vi "主程序.vi"() -> ()   [LabVIEW 2021]
uses:
  <vilib>/Utility/miscctls.llb/LVRowAndColumnTypeDef.ctl
  <vilib>/Utility/file.llb/Write Delimited Spreadsheet (string).vi
  <vilib>/Utility/file.llb/Read Delimited Spreadsheet (DBL).vi
  <instrlib>/Keithley DMM6500 DAQ6500 Series/Public/Data/Read (Single Point).vi
  <instrlib>/Keithley 27XX/Public/Data/Read Single Point.vi
  <vilib>/Utility/file.llb/Read Delimited Spreadsheet (string).vi
  <instrlib>/Keithley DMM6500 DAQ6500 Series/Keithley DMM6500 DAQ6500 Series.lvlib
  <instrlib>/Keithley 27XX/Keithley 27XX.lvlib
  <instrlib>/Keithley DMM7510/Keithley DMM7510.lvlib
panel:
  out "x*y":dbl
  in  "电压输出传感器精度":dbl(ring) items=["3‰"=0.003, "5‰"=0.005, "8‰"=0.008, "1％"=0.01, "5％"=0.05, "10％"=0.1]
  in  "量程2灵敏度":dbl(ring) items=["S12"=1.67, "S08"=2.5]
  in  "精度":dbl(ring) items=["3‰"=0.003, "5‰"=0.005, "8‰"=0.008, "1％"=0.01, "5％"=0.05, "10％"=0.1]
  out "?":bool
  in  "?":bool
  out "x != y?":bool
  in  "?":bool
  in  "SN":string
  in  "?":enum16{"CAB500", "CAB1500"}(ring)
  in  "电压读取":refnum<visa-resource-name>
  in  "仪器实例 out 4":T1
  in  "传感器缩放系数":dbl(ring) items=["2000"=2000.0, "5000"=5000.0]
  in  "量程1灵敏度":dbl(ring) items=["S12"=1.67, "S08"=2.5]
  out "?":bool
  in  "电流选择":u16(ring) items=["请选择", "5", "±100", "±200", "±300", "±50", "±500"]
  in  "?":bool
  in  "?":bool
  in  "电压输出电流传感器测试":i32(listbox)
  in  "电流传感器测试":i32(listbox)
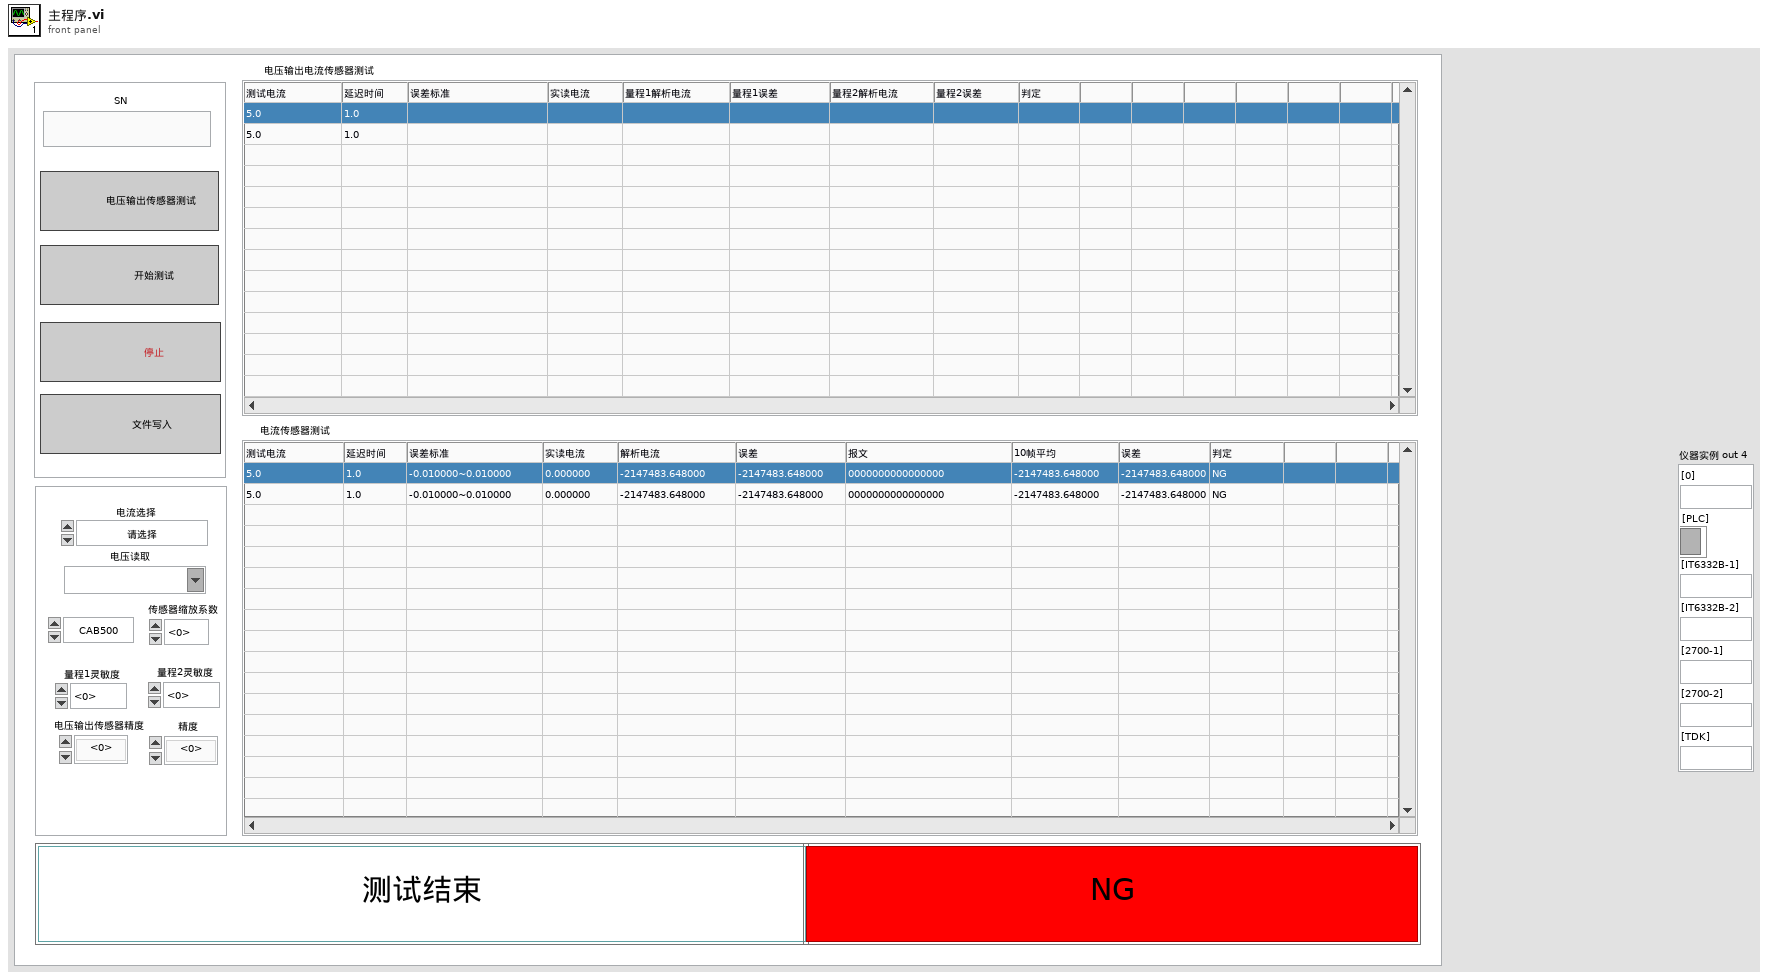
[diagram p1: front panel]
types:
  T1 = typedef "仪器实例.ctl" = cluster{"[0]":string, "[PLC]":refnum<k24>, "[IT6332B-1]":string, "[IT6332B-2]":string, "[2700-1]":string, "[2700-2]":string, "[TDK]":string}
  T2 = typedef "仪器地址输入.ctl" = cluster{"[PLC]":string, "[IT6332B-1]":string, "[IT6332B-2]":string, "[2700-1]":string, "[2700-2]":string, "[TDK]":string}
  T3 = enum16{"open", "replace", "create", "open or create", "replace or create", "replace or create with confirmation"}
  T4 = typedef "LVRowAndColumnTypeDef.ctl" = cluster{"Row":i32, "Column":i32}
  T5 = enum32{"Invalid", "Standard", "Closed", "Hidden", "Minimized", "Maximized"}
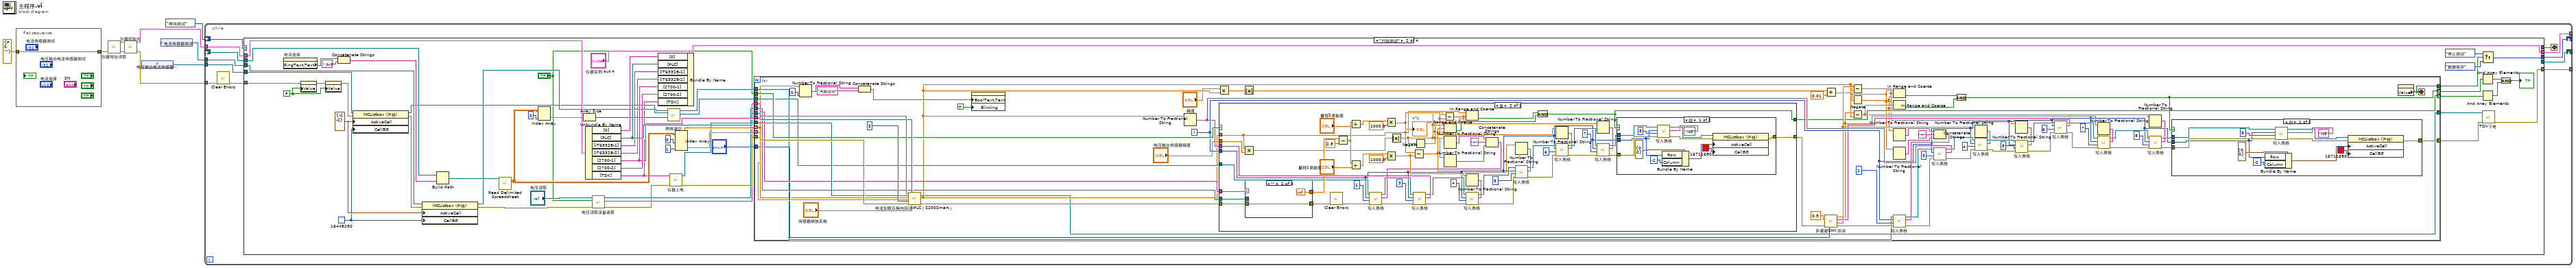
[diagram p0: block diagram]
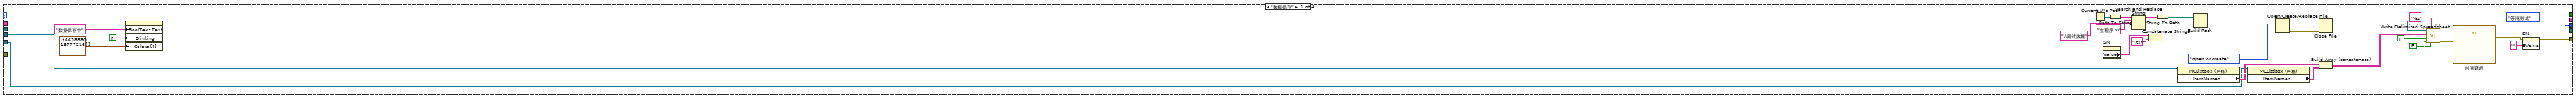
[diagram p2: hidden frame]
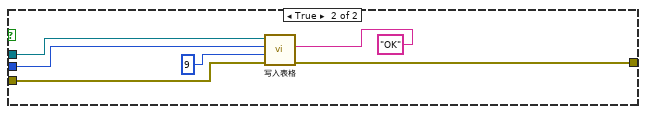
[diagram p3: hidden frame]
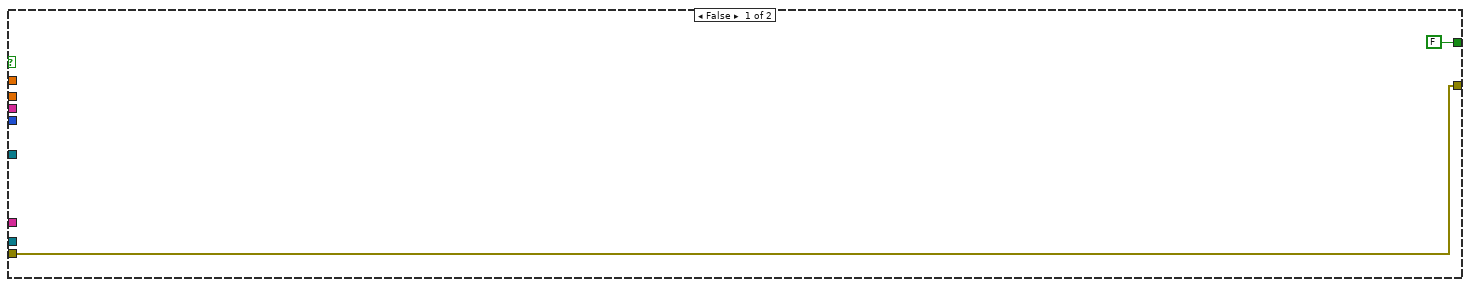
[diagram p4: hidden frame]
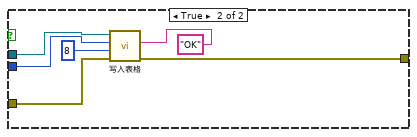
[diagram p5: hidden frame]
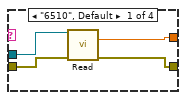
[diagram p6: hidden frame]
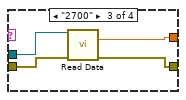
[diagram p7: hidden frame]
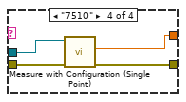
[diagram p8: hidden frame]
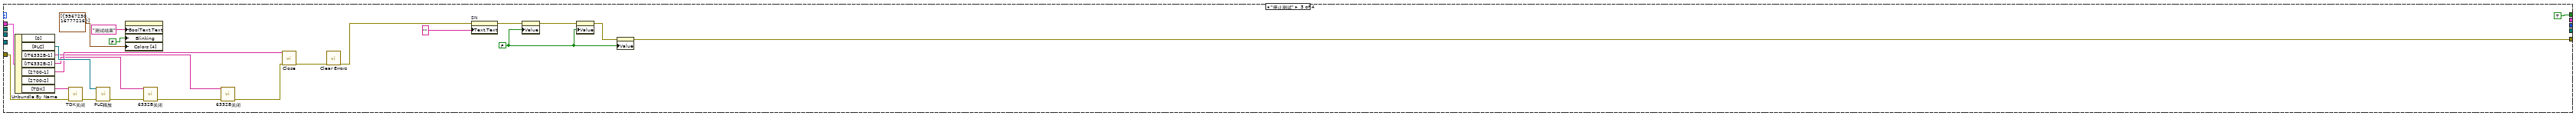
[diagram p9: hidden frame]
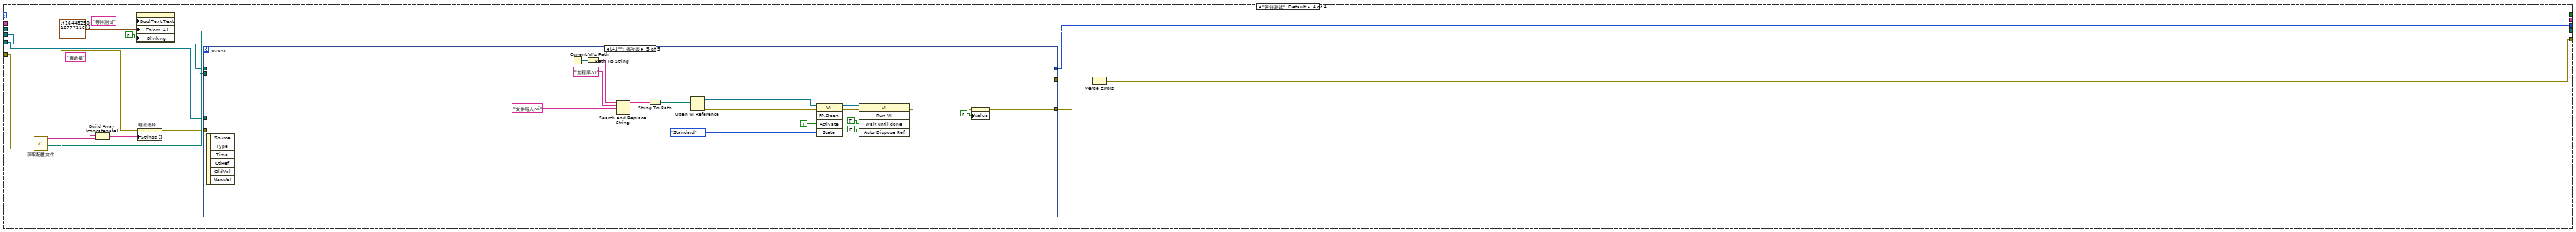
[diagram p10: hidden frame]
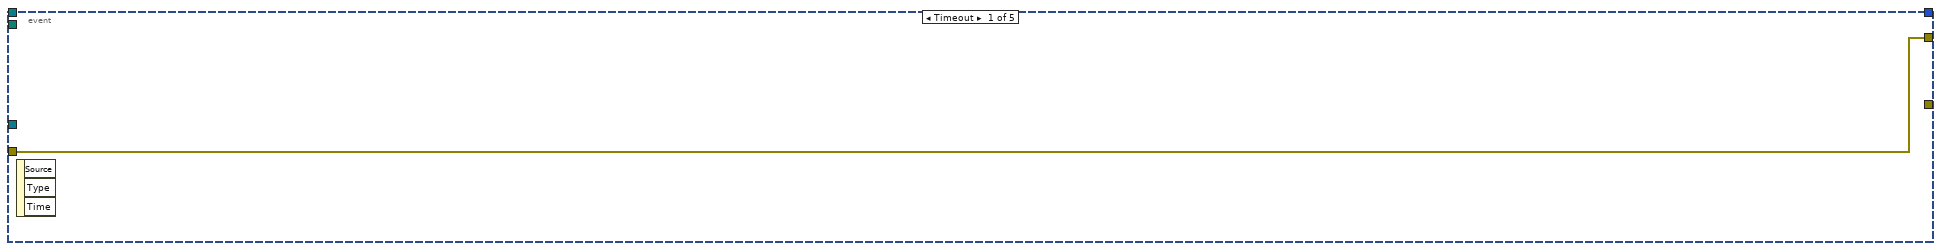
[diagram p11: hidden frame]
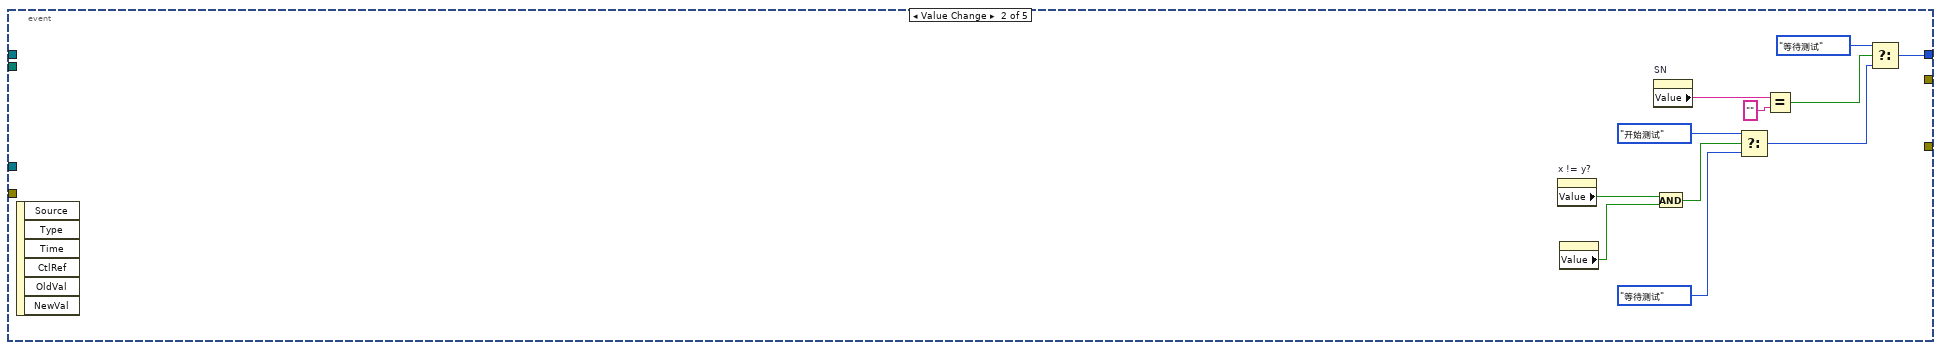
[diagram p12: hidden frame]
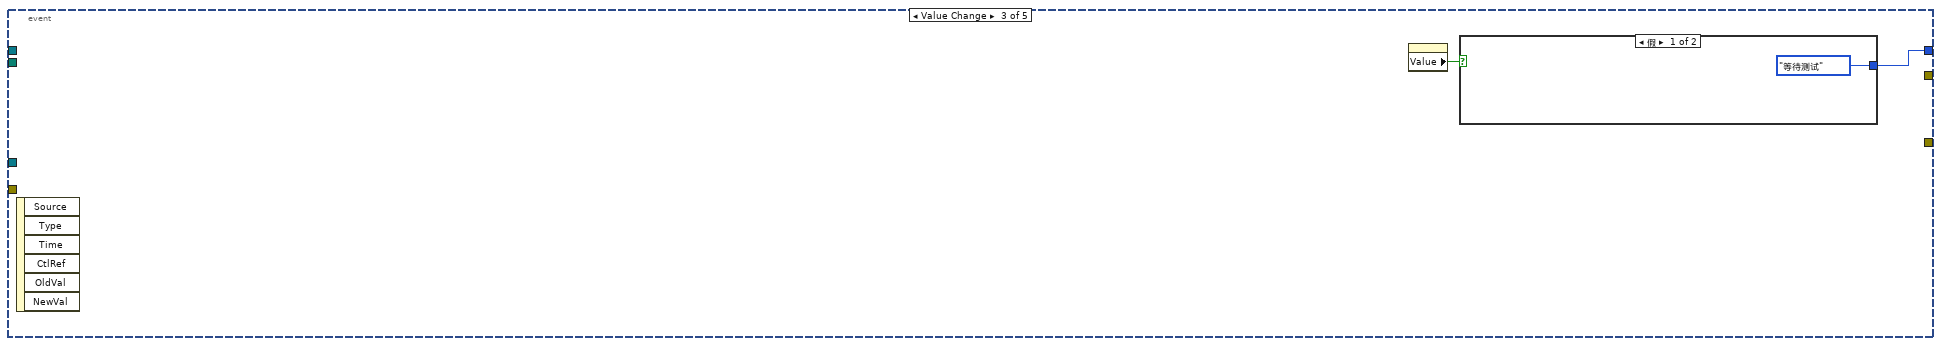
[diagram p13: hidden frame]
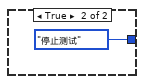
[diagram p14: hidden frame]
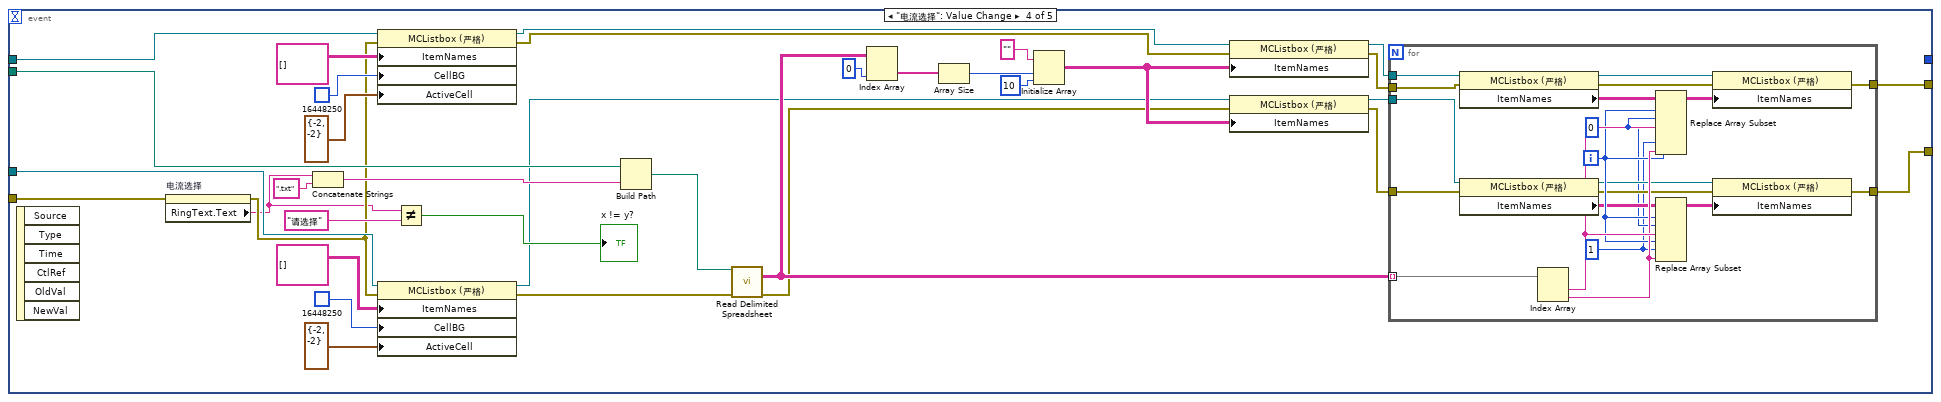
[diagram p15: hidden frame]
diagram:
  n1 = flat-sequence {
    tunnel: errorcluster {"status"=FALSE, "code"=0, "source"=""} ("error in (no error)") -> [w10]
    tunnel: [w10] -> w1
    frame #0 {
    }
  }
  n2 = call "仪器地址读取.vi"("error in (no error)"=w1) -> ("error out"=w9:errorcluster, "仪器地址"=w8:T2)  [unwired: 7 in]
  n3 = call "仪器初始化.vi"("错误输入（无错误）"=w9, "仪器地址"=w8) -> ("error out"=w6:errorcluster, "仪器实例 out"=w5:T1)  [unwired: 8 in]
  n4 = control-ref of="电压输出电流传感器测试"() -> (w3:refnum<vi>)
  n5 = control-ref of="电流传感器测试"() -> (w4:refnum<vi>)
  n6 = while {
    shift-right: [w21] -> _
    shift-left: enum16{"等待测试", "开始测试", "停止测试", "数据保存"}."等待测试" -> [w22]
    shift-right: [w17] -> _
    shift-left: _ -> [w16]
    tunnel: w3 -> [w12]
    tunnel: w4 -> [w11]
    tunnel: w5 -> [w19]
    tunnel: [w20] -> _
    tunnel: w6 -> [w14]
    tunnel: [w18] -> _
    stop <- w15 stop-if-true
    n7 = call <vilib>:"Clear Errors.vi"("error in (no error)"=w14) -> ("error out"=w13:errorcluster)  [unwired: 5 in, 1 out]
    n8 = case shown="\"开始测试\"" w22 {
      tunnel: [enum16{"等待测试", "开始测试", "停止测试", "数据保存"}."等待测试" w74 _ w319] -> w21
      tunnel: w19 -> [_ w102 w316 _]
      tunnel: w13 -> [_ w79 w312 w324]
      tunnel: [_ w101 _ _] -> w20
      tunnel: [w32 w63 w296 w325] -> w18
      tunnel: [_ _ _ w322] -> w17
      tunnel: w16 -> [_ w97 _ _]
      tunnel: [_ _ TRUE _] -> w15
      tunnel: w11 -> [w36 w89 _ w320]
      tunnel: w12 -> [w35 w90 _ w321]
      frame "数据保存" {
        n9 = property class="Bool (严格)"("BoolText.Text"="数据保存中" ("布尔文本.文本"), "Blinking"=FALSE ("闪烁"), "Colors [4]"=cluster{u32, u32}[] [{6618880, 16777216}] ("颜色[4]")) -> ()  [unwired: 2 in, 2 out]
        n10 = Current VI's Path() -> (path=w27:path)
        n11 = property on="SN" class="Str"() -> ("Value"=w34:string)  [unwired: 2 in, 2 out]
        n12 = Path To String(path=w27) -> (string=w25:string)
        n13 = Search and Replace String(input string=w25, search string="主程序.vi" ("搜索字符串"), replace string="\\测试数据" ("字符串")) -> (result string=w23:string)  [unwired: 5 in, 3 out]
        n14 = Concatenate Strings(w34, ".txt" ("字符串")) -> (w43:string)
        n15 = String To Path(string=w23) -> (path=w28:path)
        n16 = property class="MCListbox (严格)"(reference=w36) -> (error out=w54:errorcluster, "ItemNames"=w53:string[][])  [unwired: 1 in, 1 out]
        n17 = Build Path(base path=w28, name or relative path=w43) -> (appended path=w40:path)
        n18 = property class="MCListbox (严格)"(reference=w35, error in=w54) -> (error out=w48:errorcluster, "ItemNames"=w52:string[][])  [unwired: 1 out]
        n19 = Open/Create/Replace File(file path (use dialog)=w40, operation (0:open)=T3."open or create" ("操作(0:open)")) -> (refnum out=w42:refnum<file>, error out=w45:errorcluster)  [unwired: 4 in, 1 out]
        n20 = Close File(refnum=w42, error in=w45) -> (path=w39:path)  [unwired: 1 out]
        n21 = Build Array (concatenate)(w53, w52) -> (w51:string[][])
        n22 = call-poly <vilib>:"Write Delimited Spreadsheet.vi"("file path (dialog if empty)"=w39, "format (%s)"="%s", "2D data"=w51, "append to file? (new file:F)"=TRUE, "error in (no error)"=w48, "transpose? (no:F)"=FALSE) -> ("error out"=w30:errorcluster)  [unwired: 8 in, 1 out]
        n23 = call "时间延迟"("error in (no error)"=w30) -> ("error out"=w29:errorcluster)  [unwired: 10 in]
        n24 = property on="SN" class="Str"(error in=w29, "Value"="" ("SN")) -> (error out=w32:errorcluster)  [unwired: 1 in, 1 out]
      }
      frame "开始测试" {
        w81 = FALSE
        w92 = T4 {"Row"=-2, "Column"=-2} ("活动单元格:活动单元格")
        w91 = u32 16448250
        n25 = property on="电流选择" class="Ring (严格)"() -> ("RingText.Text"=w100:string)  [unwired: 2 in, 2 out]
        n26 = property class="Bool (严格)"(error in=w79, "Value"=w81) -> (error out=w82:errorcluster)  [unwired: 1 in, 1 out]
        n27 = property class="Bool (严格)"(error in=w82, "Value"=w81) -> (error out=w80:errorcluster)  [unwired: 1 in, 1 out]
        n28 = Concatenate Strings(w100, ".txt" ("字符串")) -> (w98:string)
        n29 = property class="MCListbox (严格)"(reference=w90, error in=w80, "ActiveCell"=w92, "CellBG"=w91) -> (reference out=w69:refnum<vi>, error out=w93:errorcluster)
        n30 = property class="MCListbox (严格)"(reference=w89, error in=w93, "ActiveCell"=w92, "CellBG"=w91) -> (reference out=w70:refnum<vi>, error out=w59:errorcluster)
        n31 = Build Path(base path=w97, name or relative path=w98) -> (appended path=w96:path)
        n32 = call-poly <vilib>:"Read Delimited Spreadsheet.vi"("file path (dialog if empty)"=w96) -> ("all rows"=w85:dbl[][])  [unwired: 9 in, 5 out]
        n33 = Index Array(array=w85, index (col)=0 ("禁用的索引 (列)")) -> (element=w83:dbl[])  [unwired: 1 in]
        n34 = Array Size(array=w83) -> (size(s)=w71:i32)
        n35 = Unbundle By Name(w102) -> ("[0]"=w105:string, "[PLC]"=w75:refnum<k24>, "[IT6332B-1]"=w55:string, "[IT6332B-2]"=w66:string, "[2700-1]"=w106:string, "[2700-2]"=w107:string, "[TDK]"=w67:string)
        n36 = call "电压读取设备选取.vi"("error out"=w59, "布尔"="?", "电压读取"="电压读取") -> ("error out 2"=w56:errorcluster, "所有匹配"=w57:string, "VISA resource name out"=w58:refnum<visa-resource-name>)  [unwired: 6 in]
        n37 = Bundle By Name(cluster="仪器实例 out 4", "[0]"=w105, "[PLC]"=w75, "[IT6332B-1]"=w55, "[IT6332B-2]"=w66, "[2700-1]"=w106, "[2700-2]"=w107, "[TDK]"=w67) -> (w101:T1)
        n38 = call "表格清空.vi"("数值"=w71, "电压输出电流传感器测试"=w69, "电流传感器测试"=w70) -> ("电压输出电流传感器测试 2"=w72:refnum<vi>, "电流传感器测试 2"=w73:refnum<vi>)  [unwired: 7 in]
        n39 = call "仪器上电.vi"("错误输入"=w56, "VISA resource name"=w67) -> ("error out"=w65:errorcluster, "VISA resource name out"=w68:refnum<visa-resource-name>)  [unwired: 8 in]
        n40 = Index Array(array=w85, index (col) #1=0 ("禁用的索引 (列)"), index (col) #2=1 ("索引 (列)")) -> (element #1=w110:dbl[], element #2=w109:dbl[])  [unwired: 2 in]
        n41 = for {
          tunnel: w68 -> [w181]
          tunnel: w65 -> [w185]
          tunnel: [w152] -> w64
          tunnel: w110 -> [w128] mode=indexing
          tunnel: w109 -> [w183] mode=indexing
          tunnel: w106 -> [w182]
          tunnel: w75 -> [w179]
          tunnel: w57 -> [w178]
          tunnel: w58 -> [w177]
          tunnel: "?" -> [w175]
          tunnel: "?" -> [w141]
          tunnel: w73 -> [w137]
          tunnel: w72 -> [w151]
          tunnel: [w130] -> w78 mode=indexing
          tunnel: [w129] -> w88 mode=indexing
          tunnel: [w123] -> w76
          tunnel: [w121] -> w62
          i -> [w145]
          stop <- w123 stop-if-true
          n42 = Number To Fractional String(number=w128, precision (6)=i16 0 ("精度(6)")) -> (F-format string=w132:string)  [unwired: 2 in]
          n43 = Concatenate Strings(w132, "A测试中" ("字符串")) -> (w135:string)
          n44 = call "电流加载及换向回读-PLC（S200Smart）.vi"("6510 in"=w182, "TDK in"=w181, "输入电流"=w128, "Delay Time (s)"=w183, "电源台数"=u8 3, "error in"=w185, "引用输出"=w179, "y"="传感器缩放系数") -> ("TDK out"=w121:refnum<visa-resource-name>, "实际电流"=w127:dbl, "error out"=w176:errorcluster)  [unwired: 8 in, 1 out]
          n45 = property class="Bool (严格)"("BoolText.Text"=w135, "Blinking"=TRUE ("闪烁")) -> ()  [unwired: 2 in, 2 out]
          n46 = Number To Fractional String(number=w127) -> (F-format string=w153:string)  [unwired: 3 in]
          n47 = Multiply(x="精度", y=w127) -> (x*y=w112:dbl)
          n48 = case shown="真" w175 {
            tunnel: w178 -> [_ w261]
            tunnel: w177 -> [_ w260]
            tunnel: w176 -> [w205 w259]
            tunnel: [w205 w224] -> w143
            tunnel: w153 -> [_ w253]
            tunnel: w145 -> [_ w225]
            tunnel: w127 -> [_ w220]
            tunnel: w151 -> [_ w232]
            tunnel: [FALSE w215] -> w129
            tunnel: "电压输出传感器精度" -> [_ w213]
            frame False {
            }
            frame True {
              n49 = Multiply(x=w220, y=w213) -> (x*y=w208:dbl)
              n50 = case shown="\"\"" w261 {
                tunnel: w260 -> [w283 _ w289 w290]
                tunnel: w259 -> [w281 w285 w287 w293]
                tunnel: [w280 w285 w286 w292] -> w241
                tunnel: [w282 inf w288 w291] -> w258
                frame "6510", Default {
                  n51 = call-poly <instrlib>:"Read.vi"("VISA resource name"=w283, "error in (no error)"=w281) -> ("Measurement"=w282:dbl, "error out"=w280:errorcluster)  [unwired: 11 in, 1 out]
                }
                frame "" {
                }
                frame "2700" {
                  n52 = call-poly <instrlib>:"Read Data.vi"("VISA resource name"=w289, "error in (no error)"=w287) -> ("Measurement Data"=w288:dbl, "error out"=w286:errorcluster)  [unwired: 11 in, 1 out]
                }
                frame "7510" {
                  n53 = call <instrlib>:"Measure with Configuration (Single Point).vi"("error in (no error)"=w293, "VISA resource name"=w290) -> ("error out"=w292:errorcluster, "Measurement"=w291:dbl)  [unwired: 6 in, 2 out]
                }
              }
              n54 = call <vilib>:"Clear Errors.vi"("error in (no error)"=w241) -> ("error out"=w235:errorcluster)  [unwired: 5 in, 1 out]
              n55 = Subtract(x=w258, y=2.5) -> (x-y=w222:dbl)
              n56 = Divide(x=w222, y="量程2灵敏度") -> (x/y=w219:dbl)
              n57 = Divide(x=w222, y="量程1灵敏度") -> (x/y=w255:dbl)
              n58 = Multiply(x=w219, y=1000.0) -> (x*y=w217:dbl)
              "x*y" <- w217
              n59 = Multiply(x=w255, y=1000.0) -> (x*y=w244:dbl)
              n60 = Absolute Value(x=w208) -> (abs(x)=w207:dbl)
              n61 = Subtract(x=w220, y=w244) -> (x-y=w209:dbl)
              n62 = Negate(x=w207) -> (-x=w206:dbl)
              n63 = Subtract(x=w220, y=w217) -> (x-y=w211:dbl)
              n64 = In Range and Coerce(upper limit=w207, x=w209, lower limit=w206) -> (In Range?=w212:bool)  [unwired: 1 out]
              n65 = Number To Fractional String(number=w206) -> (F-format string=w229:string)  [unwired: 3 in]
              n66 = Number To Fractional String(number=w207) -> (F-format string=w228:string)  [unwired: 3 in]
              n67 = In Range and Coerce(upper limit=w207, x=w211, lower limit=w206) -> (In Range?=w210:bool)  [unwired: 1 out]
              n68 = Number To Fractional String(number=w244) -> (F-format string=w249:string)  [unwired: 3 in]
              n69 = Concatenate Strings(w229, "~" ("字符串"), w228) -> (w227:string)
              n70 = call "写入表格.vi"("新元素/子数组"=w227, "错误输入（无错误）"=w235, "禁用的索引 (列)"=2, "索引 (行)"=w225, "引用"=w232) -> ("错误输出"=w234:errorcluster, "引用输出"=w231:refnum<vi>)  [unwired: 5 in]
              n71 = call "写入表格.vi"("新元素/子数组"=w253, "错误输入（无错误）"=w234, "禁用的索引 (列)"=3, "索引 (行)"=w225, "引用"=w231) -> ("错误输出"=w251:errorcluster, "引用输出"=w248:refnum<vi>)  [unwired: 5 in]
              n72 = call "写入表格.vi"("新元素/子数组"=w249, "错误输入（无错误）"=w251, "禁用的索引 (列)"=4, "索引 (行)"=w225, "引用"=w248) -> ("错误输出"=w250:errorcluster, "引用输出"=w247:refnum<vi>)  [unwired: 5 in]
              n73 = Number To Fractional String(number=w209) -> (F-format string=w243:string)  [unwired: 3 in]
              n74 = call "写入表格.vi"("新元素/子数组"=w243, "错误输入（无错误）"=w250, "禁用的索引 (列)"=5, "索引 (行)"=w225, "引用"=w247) -> ("错误输出"=w240:errorcluster, "引用输出"=w237:refnum<vi>)  [unwired: 5 in]
              n75 = And(x=w210, y=w212) -> (x .and. y?=w215:bool)
              n76 = Number To Fractional String(number=w217) -> (F-format string=w221:string)  [unwired: 3 in]
              n77 = call "写入表格.vi"("新元素/子数组"=w221, "错误输入（无错误）"=w240, "禁用的索引 (列)"=6, "索引 (行)"=w225, "引用"=w237) -> ("错误输出"=w239:errorcluster, "引用输出"=w236:refnum<vi>)  [unwired: 5 in]
              n78 = Number To Fractional String(number=w211) -> (F-format string=w216:string)  [unwired: 3 in]
              n79 = call "写入表格.vi"("新元素/子数组"=w216, "错误输入（无错误）"=w239, "禁用的索引 (列)"=7, "索引 (行)"=w225, "引用"=w236) -> ("错误输出"=w223:errorcluster, "引用输出"=w226:refnum<vi>)  [unwired: 5 in]
              n80 = case shown="假" w215 {
                tunnel: w223 -> [w272 w279]
                tunnel: [w267 w276] -> w224
                tunnel: w226 -> [w263 w275]
                tunnel: w225 -> [w262 w274]
                frame False {
                  n81 = call "写入表格.vi"("新元素/子数组"="NG", "错误输入（无错误）"=w272, "禁用的索引 (列)"=8, "索引 (行)"=w262, "引用"=w263) -> ("错误输出"=w268:errorcluster, "引用输出"=w271:refnum<vi>)  [unwired: 5 in]
                  n82 = Bundle By Name(cluster=T4 {"Row"=0, "Column"=0} ("活动单元格:活动单元格"), "Row"=w262, "Column"=-2) -> (w269:T4)
                  n83 = property class="MCListbox (严格)"(reference=w271, error in=w268, "ActiveCell"=w269, "CellBG"=u32 16711680) -> (error out=w267:errorcluster)  [unwired: 1 out]
                }
                frame True {
                  n84 = call "写入表格.vi"("新元素/子数组"="OK", "错误输入（无错误）"=w279, "禁用的索引 (列)"=8, "索引 (行)"=w274, "引用"=w275) -> ("错误输出"=w276:errorcluster)  [unwired: 5 in, 1 out]
                }
              }
            }
          }
          n85 = Absolute Value(x=w112) -> (abs(x)=w113:dbl)
          n86 = call "多通道CAN 回读.vi"("传感器选择"=w141, "错误输入（无错误）"=w143, "Delay Time (s)"=0.5) -> ("错误输出"=w138:errorcluster, "解析电流"=w140:dbl, "报文数组"=w125:string, "十次平均"=w139:dbl)  [unwired: 5 in]
          n87 = Add(x=w113, y=0.01) -> (x+y=w116:dbl)
          n88 = Subtract(x=w140, y=w127) -> (x-y=w117:dbl)
          n89 = Negate(x=w116) -> (-x=w115:dbl)
          n90 = Subtract(x=w139, y=w127) -> (x-y=w119:dbl)
          n91 = In Range and Coerce(upper limit=w116, x=w117, lower limit=w115) -> (In Range?=w114:bool)  [unwired: 1 out]
          n92 = In Range and Coerce(upper limit=w116, x=w119, lower limit=w115) -> (In Range?=w118:bool)  [unwired: 1 out]
          n93 = Number To Fractional String(number=w115) -> (F-format string=w147:string)  [unwired: 3 in]
          n94 = Number To Fractional String(number=w116) -> (F-format string=w149:string)  [unwired: 3 in]
          n95 = Concatenate Strings(w147, "~" ("字符串"), w149) -> (w146:string)
          n96 = call "写入表格.vi"("新元素/子数组"=w146, "错误输入（无错误）"=w138, "禁用的索引 (列)"=2, "索引 (行)"=w145, "引用"=w137) -> ("错误输出"=w150:errorcluster, "引用输出"=w136:refnum<vi>)  [unwired: 5 in]
          n97 = call "写入表格.vi"("新元素/子数组"=w153, "错误输入（无错误）"=w150, "禁用的索引 (列)"=3, "索引 (行)"=w145, "引用"=w136) -> ("错误输出"=w167:errorcluster, "引用输出"=w174:refnum<vi>)  [unwired: 5 in]
          n98 = And(x=w114, y=w118) -> (x .and. y?=w130:bool)
          n99 = Number To Fractional String(number=w140) -> (F-format string=w168:string)  [unwired: 3 in]
          n100 = call "写入表格.vi"("新元素/子数组"=w168, "错误输入（无错误）"=w167, "禁用的索引 (列)"=4, "索引 (行)"=w145, "引用"=w174) -> ("错误输出"=w166:errorcluster, "引用输出"=w173:refnum<vi>)  [unwired: 5 in]
          n101 = Number To Fractional String(number=w117) -> (F-format string=w160:string)  [unwired: 3 in]
          n102 = call "写入表格.vi"("新元素/子数组"=w160, "错误输入（无错误）"=w166, "禁用的索引 (列)"=5, "索引 (行)"=w145, "引用"=w173) -> ("错误输出"=w165:errorcluster, "引用输出"=w172:refnum<vi>)  [unwired: 5 in]
          n103 = call "写入表格.vi"("新元素/子数组"=w125, "错误输入（无错误）"=w165, "禁用的索引 (列)"=6, "索引 (行)"=w145, "引用"=w172) -> ("错误输出"=w164:errorcluster, "引用输出"=w163:refnum<vi>)  [unwired: 5 in]
          n104 = Number To Fractional String(number=w139) -> (F-format string=w162:string)  [unwired: 3 in]
          n105 = call "写入表格.vi"("新元素/子数组"=w162, "错误输入（无错误）"=w164, "禁用的索引 (列)"=7, "索引 (行)"=w145, "引用"=w163) -> ("错误输出"=w159:errorcluster, "引用输出"=w156:refnum<vi>)  [unwired: 5 in]
          n106 = Number To Fractional String(number=w119) -> (F-format string=w157:string)  [unwired: 3 in]
          n107 = call "写入表格.vi"("新元素/子数组"=w157, "错误输入（无错误）"=w159, "禁用的索引 (列)"=8, "索引 (行)"=w145, "引用"=w156) -> ("错误输出"=w155:errorcluster, "引用输出"=w154:refnum<vi>)  [unwired: 5 in]
          n108 = case shown="假" w130 {
            tunnel: w155 -> [w196 w203]
            tunnel: w154 -> [w195 w202]
            tunnel: w145 -> [w187 w200]
            tunnel: [w190 w198] -> w152
            frame False {
              n109 = Bundle By Name(cluster=T4 {"Row"=0, "Column"=0} ("活动单元格:活动单元格"), "Row"=w187, "Column"=-2) -> (w192:T4)
              n110 = call "写入表格.vi"("新元素/子数组"="NG", "错误输入（无错误）"=w196, "禁用的索引 (列)"=9, "索引 (行)"=w187, "引用"=w195) -> ("错误输出"=w191:errorcluster, "引用输出"=w194:refnum<vi>)  [unwired: 5 in]
              n111 = property class="MCListbox (严格)"(reference=w194, error in=w191, "ActiveCell"=w192, "CellBG"=u32 16711680) -> (error out=w190:errorcluster)  [unwired: 1 out]
            }
            frame True {
              n112 = call "写入表格.vi"("新元素/子数组"="OK", "错误输入（无错误）"=w203, "禁用的索引 (列)"=9, "索引 (行)"=w200, "引用"=w202) -> ("错误输出"=w198:errorcluster)  [unwired: 5 in, 1 out]
            }
          }
          n113 = property class="Bool (严格)"() -> ("Value"=w123:bool)  [unwired: 2 in, 2 out]
        }
        n114 = And Array Elements(Boolean array=w78) -> (logical AND=w87:bool)
        n115 = And Array Elements(Boolean array=w88) -> (logical AND=w86:bool)
        n116 = Select(t=enum16{"等待测试", "开始测试", "停止测试", "数据保存"}."停止测试", s=w76, f=enum16{"等待测试", "开始测试", "停止测试", "数据保存"}."数据保存") -> (s? t:f=w74:enum16{"等待测试", "开始测试", "停止测试", "数据保存"})
        n117 = call "TDK下电.vi"("error in (no error)"=w64, "VISA resource name"=w62) -> ("error out"=w63:errorcluster)  [unwired: 8 in, 1 out]
        n118 = And(x=w87, y=w86) -> (x .and. y?=→"?":bool)
      }
      frame "停止测试" {
        w300 = FALSE
        n119 = Unbundle By Name(w316) -> ("[PLC]"=w314:refnum<k24>, "[IT6332B-1]"=w306:string, "[IT6332B-2]"=w309:string, "[2700-1]"=w311:string, "[TDK]"=w315:string)  [unwired: 2 out]
        n120 = call "TDK关闭.vi"("error in (no error)"=w312, "VISA resource name"=w315) -> ("error out"=w313:errorcluster)  [unwired: 9 in]
        n121 = call "PLC释放.vi"("错误输入（无错误） 2"=w313, "引用"=w314) -> ("错误输入（无错误）"=w307:errorcluster)  [unwired: 9 in]
        n122 = property class="Bool (严格)"("BoolText.Text"="测试结束" ("布尔文本.文本"), "Blinking"=FALSE ("闪烁"), "Colors [4]"=cluster{u32, u32}[] [{9567230, 16777216}] ("颜色[4]")) -> ()  [unwired: 2 in, 2 out]
        n123 = call "6332B关闭.vi"("错误输入"=w307, "VISA资源名称"=w309) -> ("error out"=w308:errorcluster)  [unwired: 9 in]
        n124 = call "6332B关闭.vi"("错误输入"=w308, "VISA资源名称"=w306) -> ("error out"=w305:errorcluster)  [unwired: 9 in]
        n125 = call <instrlib>:"Close.vi"("VISA resource name"=w311, "error in (no error)"=w305) -> ("error out"=w295:errorcluster)  [unwired: 13 in]
        n126 = call <vilib>:"Clear Errors.vi"("error in (no error)"=w295) -> ("error out"=w294:errorcluster)  [unwired: 5 in, 1 out]
        n127 = property on="SN" class="Str"(error in=w294, "Text.Text"="" ("文本.文本")) -> (error out=w301:errorcluster)  [unwired: 1 in, 1 out]
        n128 = property class="Bool (严格)"(error in=w301, "Value"=w300) -> (error out=w303:errorcluster)  [unwired: 1 in, 1 out]
        n129 = property class="Bool (严格)"(error in=w303, "Value"=w300) -> (error out=w299:errorcluster)  [unwired: 1 in, 1 out]
        n130 = property class="Bool (严格)"(error in=w299, "Value"=w300) -> (error out=w296:errorcluster)  [unwired: 1 in, 1 out]
      }
      frame "等待测试", Default {
        n131 = call "获取配置文件.vi"("错误输入"=w324) -> ("错误输出"=w323:errorcluster, "路径输出"=w322:path, "数组"=w332:string[])  [unwired: 8 in]
        n132 = Build Array (concatenate)("请选择", w332) -> (w331:string[])
        n133 = property class="Bool (严格)"("BoolText.Text"="等待测试" ("布尔文本.文本"), "Colors [4]"=cluster{u32, u32}[] [{16448250, 16777216}] ("颜色[4]"), "Blinking"=FALSE ("闪烁")) -> ()  [unwired: 2 in, 2 out]
        n134 = property on="电流选择" class="Ring (严格)"(error in=w323, "Strings []"=w331) -> (error out=w317:errorcluster)  [unwired: 1 in, 1 out]
        n135 = event shown="[4] \"\": 值改变" {
          selector: _ -> [_ _ _ _ _]
          dyn-events: _ -> [_ _ _ _ _]
          timeout: _ -> [_ _ _ _ _]
          tunnel: [w333 _ _ w376 _] -> w327
          tunnel: [_ _ _ w375 w411] -> w326
          tunnel: w320 -> [_ _ _ w360 _]
          tunnel: w321 -> [_ _ _ w355 _]
          tunnel: w322 -> [_ _ _ w370 _]
          tunnel: [_ w337 w346 _ _] -> w319
          tunnel: w317 -> [w333 _ _ w351 _]
          event Timeout {
            n136 = event-data() -> ()  [unwired: 1 in, 3 out]
          }
          event Value Change {
            n137 = event-data() -> ()  [unwired: 1 in, 6 out]
            n138 = property on="x != y?" class="Bool (严格)"() -> ("Value"=w343:bool)  [unwired: 2 in, 2 out]
            n139 = property class="Bool (严格)"() -> ("Value"=w342:bool)  [unwired: 2 in, 2 out]
            n140 = property on="SN" class="Str"() -> ("Value"=w336:string)  [unwired: 2 in, 2 out]
            n141 = And(x=w343, y=w342) -> (x .and. y?=w344:bool)
            n142 = Select(t=enum16{"等待测试", "开始测试", "停止测试", "数据保存"}."开始测试", s=w344, f=enum16{"等待测试", "开始测试", "停止测试", "数据保存"}."等待测试") -> (s? t:f=w339:enum16{"等待测试", "开始测试", "停止测试", "数据保存"})
            n143 = Equal?(x=w336, y="") -> (x = y?=w334:bool)
            n144 = Select(t=enum16{"等待测试", "开始测试", "停止测试", "数据保存"}."等待测试", s=w334, f=w339) -> (s? t:f=w337:enum16{"等待测试", "开始测试", "停止测试", "数据保存"})
          }
          event Value Change {
            n145 = event-data() -> ()  [unwired: 1 in, 6 out]
            n146 = property class="Bool (严格)"() -> ("Value"=w345:bool)  [unwired: 2 in, 2 out]
            n147 = case shown="假" w345 {
              tunnel: [enum16{"等待测试", "开始测试", "停止测试", "数据保存"}."等待测试" enum16{"等待测试", "开始测试", "停止测试", "数据保存"}."停止测试"] -> w346
              frame False {
              }
              frame True {
              }
            }
          }
          event "电流选择": Value Change {
            n148 = event-data() -> ()  [unwired: 1 in, 6 out]
            n149 = property on="电流选择" class="Ring (严格)"(error in=w351) -> (error out=w350:errorcluster, "RingText.Text"=w349:string)  [unwired: 1 in, 1 out]
            n150 = Concatenate Strings(w349, ".txt" ("字符串")) -> (w372:string)
            n151 = property class="MCListbox (严格)"(reference=w360, error in=w350, "ItemNames"=string[][] [] ("项名"), "CellBG"=u32 16448250, "ActiveCell"=T4 {"Row"=-2, "Column"=-2} ("活动单元格:活动单元格")) -> (reference out=w359:refnum<vi>, error out=w352:errorcluster)
            n152 = property class="MCListbox (严格)"(reference=w355, error in=w350, "ItemNames"=string[][] [] ("项名"), "CellBG"=u32 16448250, "ActiveCell"=T4 {"Row"=-2, "Column"=-2} ("活动单元格:活动单元格")) -> (reference out=w354:refnum<vi>, error out=w353:errorcluster)
            n153 = Not Equal?(x=w349, y="请选择") -> (x != y?=→"x != y?":bool)
            n154 = Build Path(base path=w370, name or relative path=w372) -> (appended path=w373:path)
            n155 = call-poly <vilib>:"Read Delimited Spreadsheet.vi"("file path (dialog if empty)"=w373, "error in (no error)"=w353) -> ("all rows"=w367:string[][], "error out"=w366:errorcluster)  [unwired: 8 in, 4 out]
            n156 = Index Array(array=w367, index (col)=0 ("禁用的索引 (列)")) -> (element=w374:string[])  [unwired: 1 in]
            n157 = Array Size(array=w374) -> (size(s)=w365:i32)
            n158 = Initialize Array("", w365, 10 ("维数大小")) -> (w383:string[][])
            n159 = property class="MCListbox (严格)"(reference=w359, error in=w352, "ItemNames"=w383) -> (reference out=w380:refnum<vi>, error out=w379:errorcluster)
            n160 = property class="MCListbox (严格)"(reference=w354, error in=w366, "ItemNames"=w383) -> (reference out=w378:refnum<vi>, error out=w377:errorcluster)
            n161 = for {
              tunnel: w367 -> [w403] mode=indexing
              tunnel: w377 -> [w395]
              tunnel: w380 -> [w394]
              tunnel: w379 -> [w389]
              tunnel: [w388] -> w376
              tunnel: [w387] -> w375
              tunnel: w378 -> [w386]
              i -> [w400]
              w384 = 1 ("禁用的索引 (列)")
              w385 = 0 ("禁用的索引 (列)")
              n162 = property class="MCListbox (严格)"(reference=w394, error in=w389) -> (reference out=w391:refnum<vi>, error out=w390:errorcluster, "ItemNames"=w393:string[][])
              n163 = property class="MCListbox (严格)"(reference=w386, error in=w395) -> (reference out=w398:refnum<vi>, error out=w396:errorcluster, "ItemNames"=w399:string[][])
              n164 = Index Array(array=w403) -> (element #1=w402:string, element #2=w401:string)  [unwired: 2 in]
              n165 = Replace Array Subset(array=w393, new element #1=w402, index (row) #1=w400, index (col) #1=w385, new element #2=w401, index (row) #2=w400, index (col) #2=w384) -> (w392:string[][])
              n166 = Replace Array Subset(array=w399, new element #1=w402, index (row) #1=w400, index (col) #1=w385, new element #2=w401, index (row) #2=w400, index (col) #2=w384) -> (w397:string[][])
              n167 = property class="MCListbox (严格)"(reference=w391, error in=w390, "ItemNames"=w392) -> (error out=w388:errorcluster)  [unwired: 1 out]
              n168 = property class="MCListbox (严格)"(reference=w398, error in=w396, "ItemNames"=w397) -> (error out=w387:errorcluster)  [unwired: 1 out]
            }
          }
          event Value Change {
            n169 = event-data() -> ()  [unwired: 1 in, 6 out]
            n170 = Current VI's Path() -> (path=w409:path)
            n171 = Path To String(path=w409) -> (string=w407:string)
            n172 = Search and Replace String(input string=w407, search string="主程序.vi" ("搜索字符串"), replace string="文件写入.vi" ("字符串")) -> (result string=w404:string)  [unwired: 5 in, 3 out]
            n173 = String To Path(string=w404) -> (path=w405:path)
            n174 = Open VI Reference(vi path=w405) -> (vi reference=w420:refnum<vi>, error out=w416:errorcluster)  [unwired: 5 in]
            n175 = invoke class="VI" method="FP.Open"(reference=w420, error in=w416, "Activate"=TRUE ("激活？"), "State"=T5."Standard" ("状态")) -> (reference out=w419:refnum<vi>, error out=w415:errorcluster)  [unwired: 1 in, 3 out]
            n176 = invoke class="VI" method="Run VI"(reference=w419, error in=w415, "Wait until done"=TRUE ("结束前等待"), "Auto Dispose Ref"=FALSE ("自动销毁引用")) -> (error out=w412:errorcluster)  [unwired: 1 in, 4 out]
            n177 = property class="Bool (严格)"(error in=w412, "Value"=FALSE ("确定按钮")) -> (error out=w411:errorcluster)  [unwired: 1 in, 1 out]
          }
        }
        n178 = Merge Errors(w327, w326) -> (w325:errorcluster)
      }
    }
  }
